vi "TEG_info_show.vi"() -> ()   [LabVIEW 2021]
panel:
  out "DT ref":string="0 ºC"
  out "TC OUT":T1={"Hot"="0 ºC", "Cold"="0 ºC", "Diff"="0 ºC"}
  out "gas temp DT":string="0 ºC"
  out "TC IN":T1={"Hot"="0 ºC", "Cold"="0 ºC", "Diff"="0 ºC"}
  out "gas temp in":string="0 ºC"
  out "gas temp out":string="0 ºC"
  out "ref H":string="0 ºC"
  out "ref C":string="0 ºC"
  out "DT ref 2":string="0 ºC"
  out "TC OUT 2":T1={"Hot"="0 ºC", "Cold"="0 ºC", "Diff"="0 ºC"}
  out "gas temp DT 2":string="0 ºC"
  out "TC IN 2":T1={"Hot"="0 ºC", "Cold"="0 ºC", "Diff"="0 ºC"}
  out "gas temp in 2":string="0 ºC"
  out "gas temp out 2":string="0 ºC"
  out "ref H 2":string="0 ºC"
  out "ref C 2":string="0 ºC"
  in  "stop":bool
  # "HIGH TEMPERATURE TEG"
  # "DT"
  # "DT"
  # "LOW TEMPERATURE TEG"
  # "DT"
  # "DT"
  # "DT"
  # "HOT SIDE"
  # "COLD SIDE"
  # "DT"
  # "HOT SIDE"
  # "COLD SIDE"
  # "DT"
  # "HOT SIDE"
  # "COLD SIDE"
  # "DT"
  # "HOT SIDE"
  # "COLD SIDE"
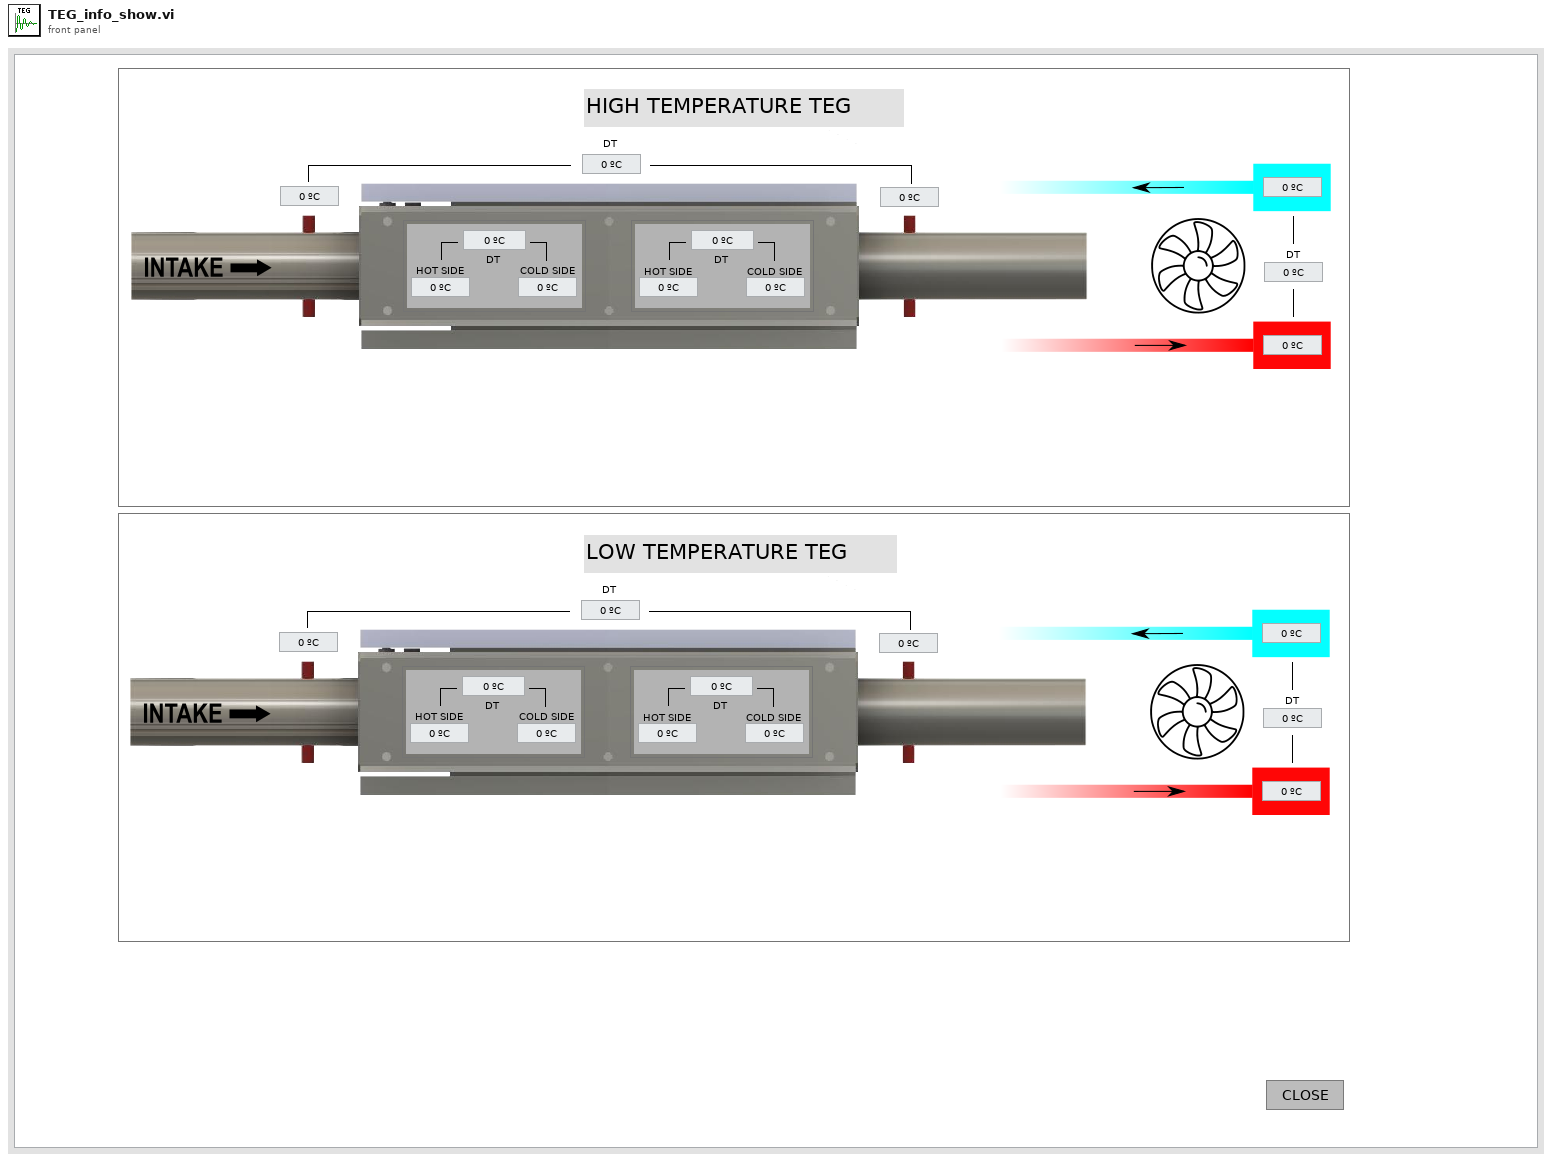
[diagram p1: front panel]
types:
  T1 = cluster{"Hot":string, "Cold":string, "Diff":string}
  T2 = cluster{"ValvePos1":sgl, "ValvePos2":sgl, "PressureArray":sgl[], "TempArray2":sgl[], "TempArray1":sgl[], "Time Stamp":timestamp}[]
  T3 = cluster{"ValvePos1":sgl, "ValvePos2":sgl, "PressureArray":sgl[], "TempArray2":sgl[], "TempArray1":sgl[], "Time Stamp":timestamp}
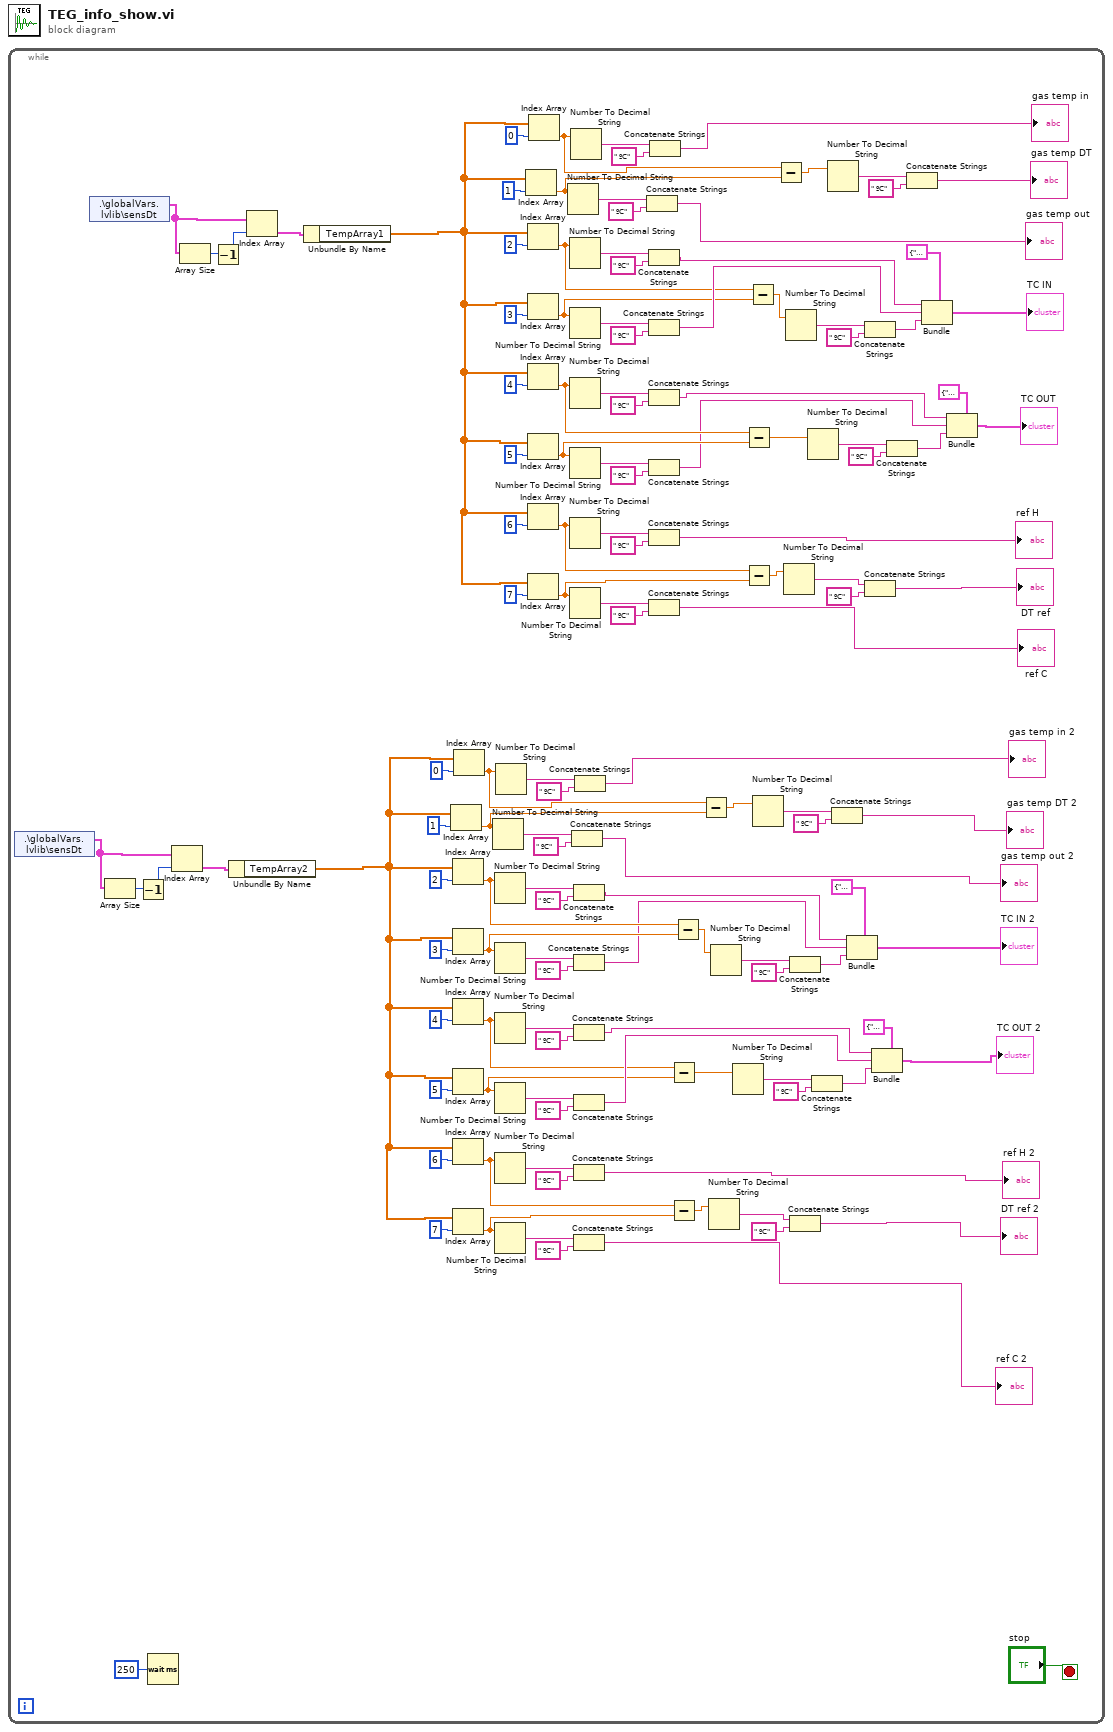
[diagram p0: block diagram]
diagram:
  n1 = while {
    stop <- "stop" stop-if-true
    n2 = shared-variable ".\\globalVars.lvlib\\sensDt"() -> (w63:T2)  [unwired: 1 in, 1 out]
    n3 = shared-variable ".\\globalVars.lvlib\\sensDt"() -> (w68:T2)  [unwired: 1 in, 1 out]
    n4 = Array Size(array=w63) -> (size(s)=w33:i32)
    n5 = Decrement(x=w33) -> (x-1=w34:i32)
    n6 = Wait (ms)(milliseconds to wait=u32 250) -> ()  [unwired: 1 out]
    n7 = Index Array(array=w63, index=w34) -> (element=w64:T3)
    n8 = Array Size(array=w68) -> (size(s)=w104:i32)
    n9 = Decrement(x=w104) -> (x-1=w103:i32)
    n10 = Unbundle By Name(w64) -> ("TempArray2"=w65:sgl[])
    n11 = Index Array(array=w68, index=w103) -> (element=w67:T3)
    n12 = Unbundle By Name(w67) -> ("TempArray1"=w66:sgl[])
    n13 = Index Array(array=w65, index=1) -> (element=w55:sgl)
    n14 = Index Array(array=w65, index=2) -> (element=w56:sgl)
    n15 = Index Array(array=w65, index=3) -> (element=w57:sgl)
    n16 = Index Array(array=w65, index=4) -> (element=w39:sgl)
    n17 = Index Array(array=w65, index=5) -> (element=w40:sgl)
    n18 = Index Array(array=w65, index=6) -> (element=w50:sgl)
    n19 = Index Array(array=w65, index=7) -> (element=w51:sgl)
    n20 = Index Array(array=w65, index=0) -> (element=w54:sgl)
    n21 = Number To Decimal String(number=w55) -> (decimal integer string=w11:string)  [unwired: 1 in]
    n22 = Number To Decimal String(number=w56) -> (decimal integer string=w13:string)  [unwired: 1 in]
    n23 = Number To Decimal String(number=w57) -> (decimal integer string=w15:string)  [unwired: 1 in]
    n24 = Number To Decimal String(number=w39) -> (decimal integer string=w17:string)  [unwired: 1 in]
    n25 = Number To Decimal String(number=w40) -> (decimal integer string=w19:string)  [unwired: 1 in]
    n26 = Number To Decimal String(number=w50) -> (decimal integer string=w21:string)  [unwired: 1 in]
    n27 = Number To Decimal String(number=w51) -> (decimal integer string=w23:string)  [unwired: 1 in]
    n28 = Number To Decimal String(number=w54) -> (decimal integer string=w9:string)  [unwired: 1 in]
    n29 = Index Array(array=w66, index=1) -> (element=w76:sgl)
    n30 = Index Array(array=w66, index=2) -> (element=w75:sgl)
    n31 = Index Array(array=w66, index=3) -> (element=w74:sgl)
    n32 = Index Array(array=w66, index=4) -> (element=w96:sgl)
    n33 = Index Array(array=w66, index=5) -> (element=w95:sgl)
    n34 = Index Array(array=w66, index=6) -> (element=w82:sgl)
    n35 = Index Array(array=w66, index=7) -> (element=w81:sgl)
    n36 = Index Array(array=w66, index=0) -> (element=w77:sgl)
    n37 = Number To Decimal String(number=w76) -> (decimal integer string=w126:string)  [unwired: 1 in]
    n38 = Number To Decimal String(number=w75) -> (decimal integer string=w124:string)  [unwired: 1 in]
    n39 = Number To Decimal String(number=w74) -> (decimal integer string=w122:string)  [unwired: 1 in]
    n40 = Number To Decimal String(number=w96) -> (decimal integer string=w120:string)  [unwired: 1 in]
    n41 = Number To Decimal String(number=w95) -> (decimal integer string=w118:string)  [unwired: 1 in]
    n42 = Number To Decimal String(number=w82) -> (decimal integer string=w116:string)  [unwired: 1 in]
    n43 = Number To Decimal String(number=w81) -> (decimal integer string=w114:string)  [unwired: 1 in]
    n44 = Number To Decimal String(number=w77) -> (decimal integer string=w128:string)  [unwired: 1 in]
    n45 = Concatenate Strings(w11, " ºC") -> (→"gas temp out 2":string)
    n46 = Concatenate Strings(w13, " ºC") -> (w43:string)
    n47 = Concatenate Strings(w15, " ºC") -> (w44:string)
    n48 = Concatenate Strings(w17, " ºC") -> (w46:string)
    n49 = Concatenate Strings(w19, " ºC") -> (w47:string)
    n50 = Concatenate Strings(w21, " ºC") -> (→"ref H 2":string)
    n51 = Concatenate Strings(w23, " ºC") -> (→"ref C 2":string)
    n52 = Concatenate Strings(w9, " ºC") -> (→"gas temp in 2":string)
    n53 = Concatenate Strings(w126, " ºC") -> (→"gas temp out":string)
    n54 = Concatenate Strings(w124, " ºC") -> (w91:string)
    n55 = Concatenate Strings(w122, " ºC") -> (w90:string)
    n56 = Concatenate Strings(w120, " ºC") -> (w88:string)
    n57 = Concatenate Strings(w118, " ºC") -> (w87:string)
    n58 = Concatenate Strings(w116, " ºC") -> (→"ref H":string)
    n59 = Concatenate Strings(w114, " ºC") -> (→"ref C":string)
    n60 = Concatenate Strings(w128, " ºC") -> (→"gas temp in":string)
    n61 = Subtract(x=w39, y=w40) -> (x-y=w59:sgl)
    n62 = Subtract(x=w50, y=w51) -> (x-y=w61:sgl)
    n63 = Subtract(x=w56, y=w57) -> (x-y=w58:sgl)
    n64 = Subtract(x=w54, y=w55) -> (x-y=w60:sgl)
    n65 = Number To Decimal String(number=w61) -> (decimal integer string=w62:string)  [unwired: 1 in]
    n66 = Number To Decimal String(number=w58) -> (decimal integer string=w35:string)  [unwired: 1 in]
    n67 = Number To Decimal String(number=w59) -> (decimal integer string=w38:string)  [unwired: 1 in]
    n68 = Subtract(x=w96, y=w95) -> (x-y=w72:sgl)
    n69 = Subtract(x=w82, y=w81) -> (x-y=w70:sgl)
    n70 = Subtract(x=w75, y=w74) -> (x-y=w73:sgl)
    n71 = Number To Decimal String(number=w60) -> (decimal integer string=w52:string)  [unwired: 1 in]
    n72 = Subtract(x=w77, y=w76) -> (x-y=w71:sgl)
    n73 = Number To Decimal String(number=w70) -> (decimal integer string=w69:string)  [unwired: 1 in]
    n74 = Number To Decimal String(number=w73) -> (decimal integer string=w100:string)  [unwired: 1 in]
    n75 = Concatenate Strings(w35, " ºC") -> (w45:string)
    n76 = Concatenate Strings(w62, " ºC") -> (→"DT ref 2":string)
    n77 = Number To Decimal String(number=w72) -> (decimal integer string=w97:string)  [unwired: 1 in]
    n78 = Concatenate Strings(w38, " ºC") -> (w48:string)
    n79 = Number To Decimal String(number=w71) -> (decimal integer string=w80:string)  [unwired: 1 in]
    n80 = Concatenate Strings(w52, " ºC") -> (→"gas temp DT 2":string)
    n81 = Bundle(cluster=T1 {"Hot"="", "Cold"="", "Diff"=""}, "Hot"=w43, "Cold"=w44, "Diff"=w45) -> (→"TC IN 2":T1)
    n82 = Concatenate Strings(w100, " ºC") -> (w89:string)
    n83 = Concatenate Strings(w69, " ºC") -> (→"DT ref":string)
    n84 = Bundle(cluster=T1 {"Hot"="", "Cold"="", "Diff"=""}, "Hot"=w46, "Cold"=w47, "Diff"=w48) -> (→"TC OUT 2":T1)
    n85 = Concatenate Strings(w97, " ºC") -> (w86:string)
    n86 = Concatenate Strings(w80, " ºC") -> (→"gas temp DT":string)
    n87 = Bundle(cluster=T1 {"Hot"="", "Cold"="", "Diff"=""}, "Hot"=w91, "Cold"=w90, "Diff"=w89) -> (→"TC IN":T1)
    n88 = Bundle(cluster=T1 {"Hot"="", "Cold"="", "Diff"=""}, "Hot"=w88, "Cold"=w87, "Diff"=w86) -> (→"TC OUT":T1)
  }
